vi "Populate gRPC Events.vi"(7 "RPC Method Parameters":T1[](array[typedef]), 8 "error in (no error)":errorcluster, 10 "Server class in":refnum<vi>, 11 "Server library in":refnum<vi>) -> (0 "error out":errorcluster, 2 "Server class out":refnum<vi>, 3 "Server library out":refnum<vi>)   [LabVIEW 2019, in "gRPC Scripting Tools.lvlib"]
uses:
  gRPC Scripting Tools.lvlib
  TypeDefs/RPC Method Parameters.ctl
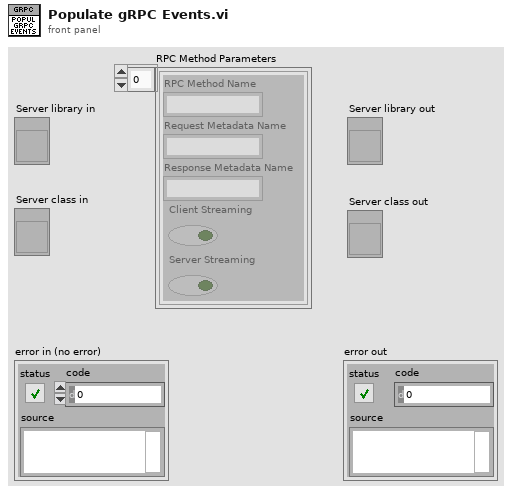
[diagram p1: front panel]
types:
  T1 = typedef "gRPC Scripting Tools.lvlib/RPC Method Parameters.ctl" = cluster{"RPC Method Name":string, "Request Metadata Name":string, "Response Metadata Name":string, "Client Streaming":bool, "Server Streaming":bool}
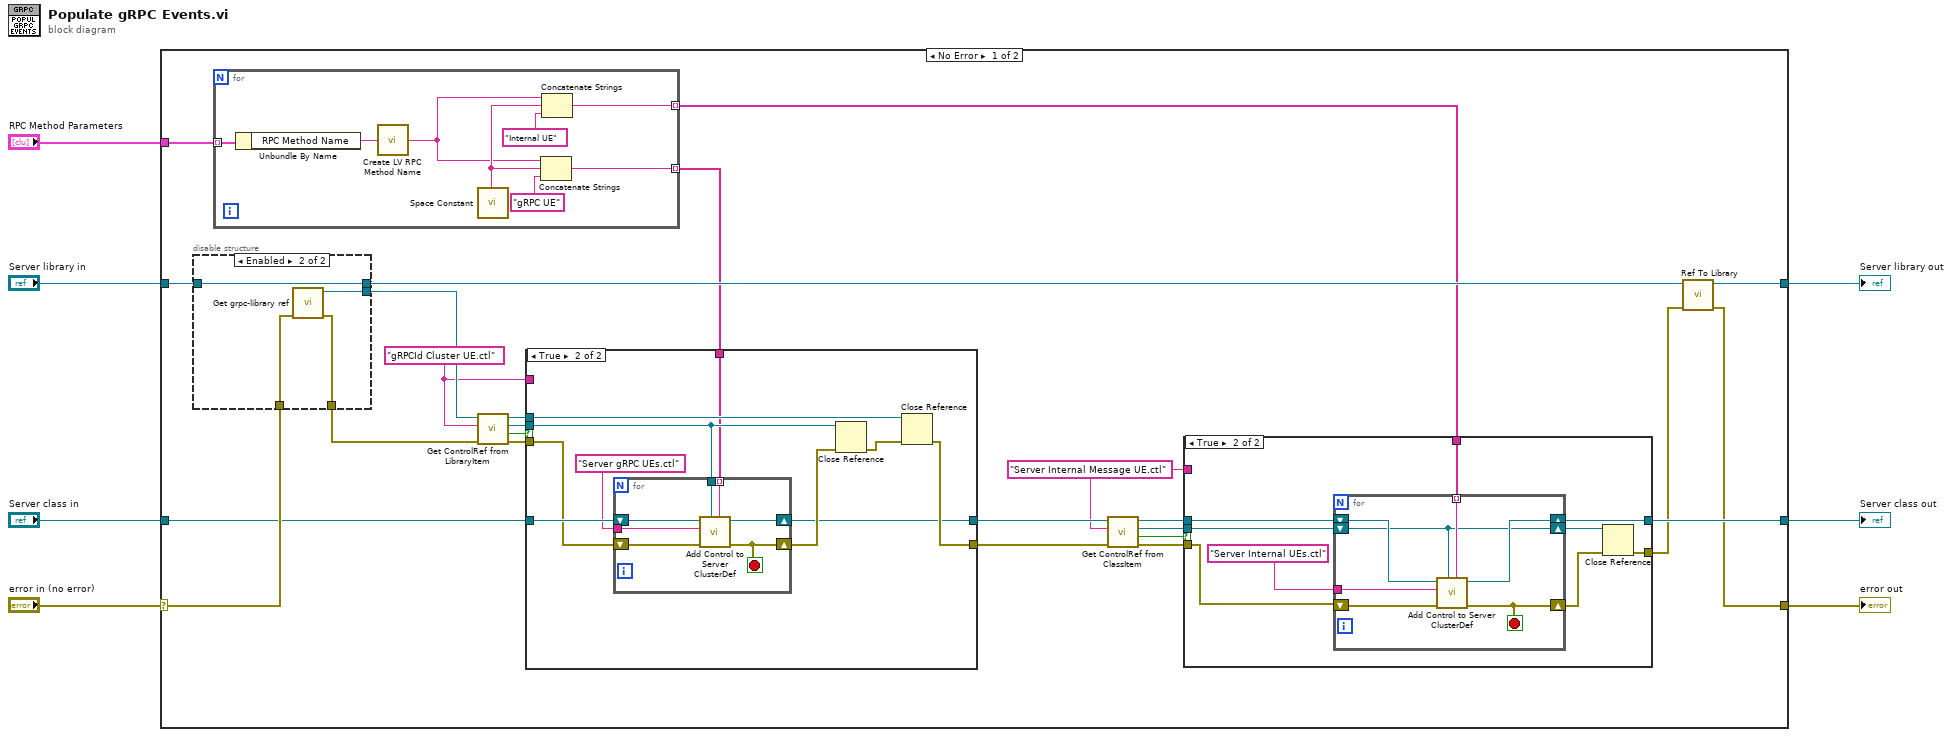
[diagram p0: block diagram]
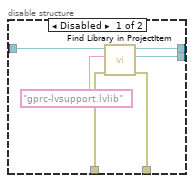
[diagram p2: hidden frame]
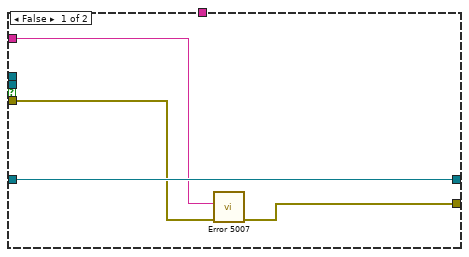
[diagram p3: hidden frame]
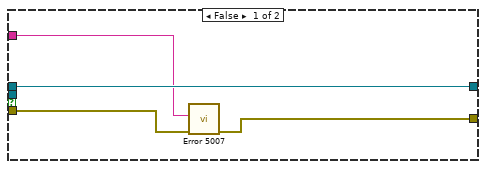
[diagram p4: hidden frame]
diagram:
  n1 = case shown="No Error" "error in (no error)" {
    selector: "error in (no error)" -> [w20 w92]
    tunnel: [w17 w92] -> w7
    tunnel: [w32 w94] -> w6
    tunnel: [w18 w93] -> w2
    tunnel: "Server class in" -> [w8 w94]
    tunnel: "Server library in" -> [w30 w93]
    tunnel: "RPC Method Parameters" -> [w16 _]
    frame No Error {
      w11 = "Server Internal Message UE.ctl" ("Item Name")
      w9 = "gRPCId Cluster UE.ctl" ("y")
      n2 = disable-structure shown="Enabled" {
        disable-tunnel: w30 -> [w38 w42]
        disable-tunnel: [w37 w39] -> w22
        disable-tunnel: [w36 w41] -> w21
        disable-tunnel: w20 -> [w34 w40]
        disable-tunnel: [w33 w42] -> w19
        frame Disabled {
          n3 = call "Find Library in ProjectItem.vi"("error in (no error)"=w34, "Library Name"="gprc-lvsupport.lvlib", "ProjectItem in"=w38) -> ("error out"=w37:errorcluster, "Library out"=w36:refnum<vi>, "ProjectItem out"=w33:refnum<vi>)  [unwired: 5 in, 1 out]
        }
        frame Enabled {
          n4 = call "Get grpc-library ref.vi"("error in"=w40) -> ("error out"=w39:errorcluster, "Library out"=w41:refnum<vi>)  [unwired: 9 in]
        }
      }
      n5 = for {
        tunnel: w16 -> [w91] mode=indexing
        tunnel: [w89] -> w15 mode=indexing
        tunnel: [w87] -> w14 mode=indexing
        n6 = Unbundle By Name(w91) -> ("RPC Method Name"=w85:string)
        n7 = call "Create LV RPC Method Name.vi"("Proto Parser RPC Method Name in"=w85) -> ("LV RPC Method Name out"=w84:string)
        n8 = call <vilib>:"Space Constant.vi"() -> ("String"=w86:string)
        n9 = Concatenate Strings(w84, w86, "gRPC UE" ("string")) -> (w89:string)
        n10 = Concatenate Strings(w84, w86, "Internal UE" ("string")) -> (w87:string)
      }
      n11 = call "Get ControlRef from LibraryItem.vi"("error in (no error)"=w22, "Control Name"=w9, "Library item in"=w21) -> ("error out"=w29:errorcluster, "Found?"=w10:bool, "Control ref out"=w27:refnum<vi>, "Library item out"=w28:refnum<vi>)  [unwired: 5 in]
      n12 = case shown="True" w10 {
        tunnel: [w43 w56] -> w31
        tunnel: w8 -> [w46 w55]
        tunnel: w29 -> [w45 w54]
        tunnel: w28 -> [_ w53]
        tunnel: w27 -> [_ w51]
        tunnel: [w46 w49] -> w23
        tunnel: w15 -> [_ w47]
        tunnel: w9 -> [w44 _]
        frame False {
          n13 = call "Error 5007.vi"("error in (no error)"=w45, "Target ClusterDef Name"=w44) -> ("error out"=w43:errorcluster)  [unwired: 9 in]
        }
        frame True {
          n14 = for {
            tunnel: "Server gRPC UEs.ctl" ("Item Name") -> [w61]
            tunnel: w51 -> [w60]
            shift-right: [w57] -> w50
            shift-left: w54 -> [w63]
            tunnel: w47 -> [w59] mode=indexing
            shift-right: [w58] -> w49
            shift-left: w55 -> [w62]
            stop <- w57 stop-if-true
            n15 = call "Add Control to Server ClusterDef.vi"("New Control Label"=w59, "Source Control ref in"=w60, "error in (no error)"=w63, "Target ClusterDef Name"=w61, "Server class in"=w62) -> ("error out"=w57:errorcluster, "Server class out"=w58:refnum<vi>)  [unwired: 5 in]
          }
          n16 = Close Reference(reference=w51, error in (no error)=w50) -> (error out=w52:errorcluster)
          n17 = Close Reference(reference=w53, error in (no error)=w52) -> (error out=w56:errorcluster)
        }
      }
      n18 = call "Get ControlRef from ClassItem.vi"("error in (no error)"=w31, "Item Name"=w11, "LVClassLibrary in"=w23) -> ("error out"=w25:errorcluster, "Found ?"=w12:bool, "Control ref out"=w26:refnum<vi>, "LVClassLibrary out"=w24:refnum<vi>)  [unwired: 5 in]
      n19 = case shown="True" w12 {
        tunnel: [w67 w76] -> w32
        tunnel: w26 -> [_ w75]
        tunnel: w25 -> [w66 w74]
        tunnel: w24 -> [w67 w73]
        tunnel: w14 -> [_ w71]
        tunnel: [w65 w68] -> w13
        tunnel: w11 -> [w64 _]
        frame False {
          n20 = call "Error 5007.vi"("error in (no error)"=w66, "Target ClusterDef Name"=w64) -> ("error out"=w65:errorcluster)  [unwired: 9 in]
        }
        frame True {
          n21 = for {
            tunnel: "Server Internal UEs.ctl" ("Target ClusterDef Name") -> [w81]
            tunnel: w71 -> [w80] mode=indexing
            shift-right: [w79] -> w76
            shift-left: w73 -> [w82]
            shift-right: [w78] -> w70
            shift-left: w74 -> [w83]
            shift-right: [w77] -> w69
            shift-left: w75 -> [w77]
            stop <- w78 stop-if-true
            n22 = call "Add Control to Server ClusterDef.vi"("New Control Label"=w80, "Source Control ref in"=w77, "error in (no error)"=w83, "Target ClusterDef Name"=w81, "Server class in"=w82) -> ("error out"=w78:errorcluster, "Server class out"=w79:refnum<vi>)  [unwired: 5 in]
          }
          n23 = Close Reference(reference=w69, error in (no error)=w70) -> (error out=w68:errorcluster)
        }
      }
      n24 = call "Ref To Library.vi"("error in (no error)"=w13, "ProjectItem in"=w19) -> ("error out"=w17:errorcluster, "Library out"=w18:refnum<vi>)  [unwired: 8 in]
    }
    frame Error {
    }
  }
  "error out" <- w7
  "Server class out" <- w6
  "Server library out" <- w2
